vi "getBubblesStd.vi"(3 "Circles Data in":T2(array[cluster])) -> (0 "Plot mean":dbl(graph), 1 "bubbleFeatures":T1, 2 "Plot SD":dbl(graph))   [LabVIEW 2013]
uses:
  <vilib>/Analysis/NI_AALBase.lvlib
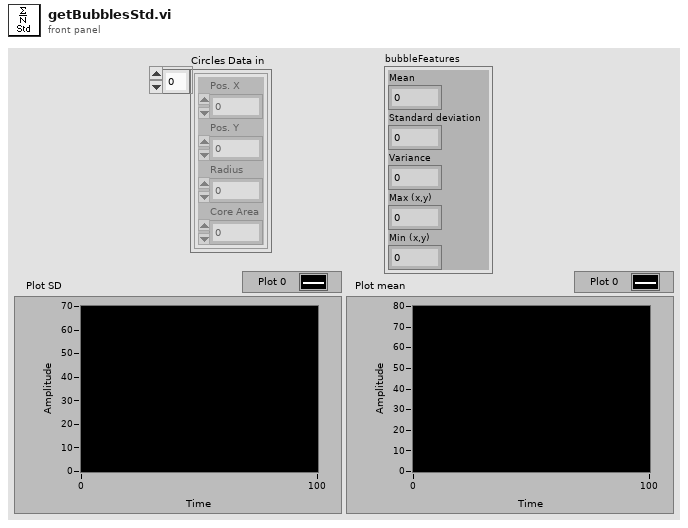
[diagram p1: front panel]
types:
  T1 = cluster{"Mean":dbl, "Standard deviation":dbl, "Variance":dbl, "Max (x,y)":dbl, "Min (x,y)":dbl}
  T2 = cluster{"Pos. X":i32, "Pos. Y":i32, "Radius":i32, "Core Area":i32}[]
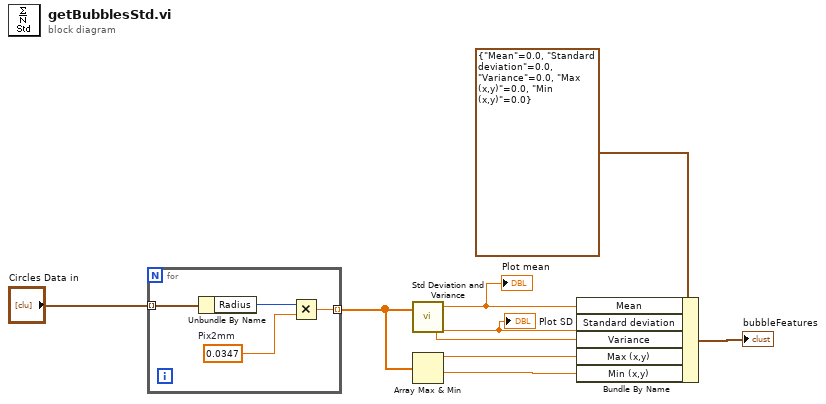
[diagram p0: block diagram]
diagram:
  n1 = for {
    tunnel: "Circles Data in" -> [w13] mode=indexing
    tunnel: [w10] -> w8 mode=indexing
    w11 = 0.0347  # Pix2mm
    n2 = Unbundle By Name(w13) -> ("Radius"=w12:i32)
    n3 = Multiply(x=w12, y=w11) -> (x*y=w10:dbl)
  }
  n4 = call <vilib>:"Std Deviation and Variance.vi"("X"=w8) -> ("mean"=w2:dbl, "standard deviation"=w1:dbl, "variance"=w6:dbl)  [unwired: 1 in]
  "Plot SD" <- w1
  "Plot mean" <- w2
  n5 = Array Max & Min(array=w8) -> (max value=w5:dbl, min value=w4:dbl)  [unwired: 2 out]
  n6 = Bundle By Name(cluster=T1 {"Mean"=0.0, "Standard deviation"=0.0, "Variance"=0.0, "Max (x,y)"=0.0, "Min (x,y)"=0.0}, "Mean"=w2, "Standard deviation"=w1, "Variance"=w6, "Max (x,y)"=w5, "Min (x,y)"=w4) -> (→"bubbleFeatures":T1)
